vi "DDS Wake Up.vi"(8 "error in (no error)":errorcluster, 10 "chanel number (1)":u8=1 min=1 max=4 step=1, 11 "DDS ref in":T1={"NI USB-8451 device reference"="", "DIO port"=0, "Serial Clock Rate [kHz]"=1000}) -> (0 "error out":errorcluster, 3 "DDS ref out":T1={"NI USB-8451 device reference"="", "DIO port"=0, "Serial Clock Rate [kHz]"=1000})   [LabVIEW 2013, in "DDS.lvlib"]
doc: "Wakes up the specified channel from a DDS Power Down command, restoring its previous state without erasing data."
uses:
  DDS.lvlib
  Controls/DDS Box Device Reference.ctl
  <vilib>/ni845x/ni845x.llb/ni845xControl.ctl
  Controls/AD9910 registers.ctl
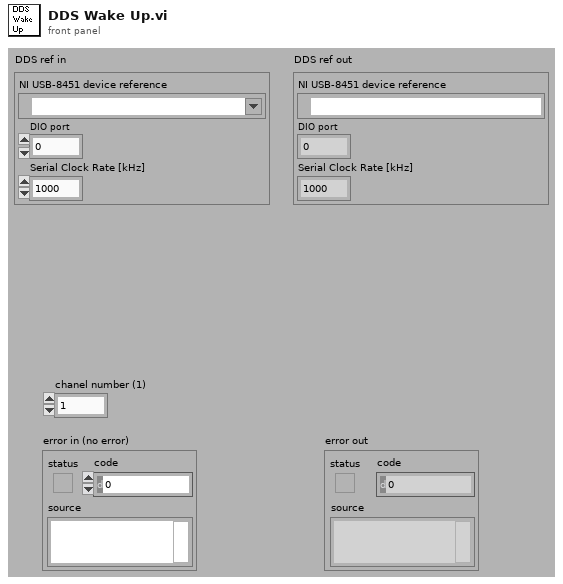
[diagram p1: front panel]
types:
  T1 = typedef "DDS.lvlib/DDS Box Device Reference.ctl" = cluster{"NI USB-8451 device reference":T2, "DIO port":u8, "Serial Clock Rate [kHz]":u16}
  T2 = typedef "ni845xControl.ctl" = refnum<k21>
  T3 = typedef "DDS.lvlib/AD9910 registers.ctl" = enum16{"CFR1", "CFR2", "CFR3", "Auxiliary DAC Control", "I/0 Update Rate", "Frequency Tuning Word", "Phase Offset Word", "Amplitude Scale Factor", "Multichip Sync", "Digital Ramp Limit", "Digital Ramp Step Size", "Digital Ramp Rate", "Single Tone Profile 0", "Single Tone Profile 1", "Single Tone Profile 2", "Single Tone Profile 3", "Single Tone Profile 4", "Single Tone Profile 5", "Single Tone Profile 6", "Single Tone Profile 7", "RAM Profile 0", "RAM Profile 1", "RAM Profile 2", "RAM Profile 3", "RAM Profile 4", "RAM Profile 5", "RAM Profile 6", "RAM Profile 7", "RAM"}
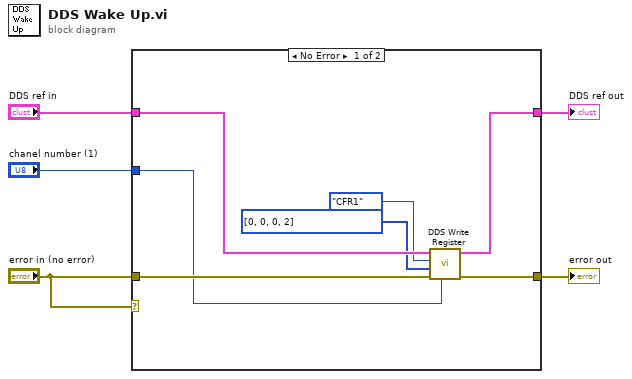
[diagram p0: block diagram]
diagram:
  n1 = case shown="No Error" "error in (no error)" {
    tunnel: "error in (no error)" -> [w7 w13]
    tunnel: "DDS ref in" -> [w12 w14]
    tunnel: [w9 w14] -> w3
    tunnel: [w8 w13] -> w2
    tunnel: "chanel number (1)" -> [w6 _]
    frame No Error {
      n2 = call "DDS Write Register.vi"("channel number (1)"=w6, "error in (no error)"=w7, "Write Data"=u8[] [0, 0, 0, 2], "Register"=AD9910_registers."CFR1", "DDS ref in"=w12) -> ("error out"=w8:errorcluster, "DDS ref out"=w9:T1)  [unwired: 4 in, 1 out]
    }
    frame Error {
    }
  }
  "error out" <- w2
  "DDS ref out" <- w3
